vi "IR GALVO CONTROL (MULTI SPOT).vi"() -> ()   [LabVIEW 2015]
uses:
  <vilib>/DAQmx/write.llb/DAQmx Write (Analog 2D DBL NChan NSamp).vi
  <vilib>/DAQmx/configure/timing.llb/DAQmx Timing (Sample Clock).vi
  <vilib>/DAQmx/miscellaneous.llb/DAQmx Fill In Error Info.vi
panel:
  in  "Stop Button":bool
  in  "Cycle Time (ms)":i32=50
  in  "IR Stimulus Settings":cluster{"X":dbl, "Y":dbl, "TON (ms)":dbl}[](array[cluster])=[{"X"=600.0, "Y"=600.0, "TON (ms)"=12.5}, {"X"=1200.0, "Y"=1200.0, "TON (ms)"=12.5}, {"X"=1800.0, "Y"=1800.0, "TON (ms)"=12.5}, {"X"=2400.0, "Y"=2400.0, "TON (ms)"=12.5}] {"TON (ms)" step=0.1 format="%#.1f"; "Y" step=1.0 format="%#.0f"; "X" step=1.0 format="%#.0f"}
  in  "DAQmx Task Name":refnum<k21>="GALVO 1"
  out "Stim Count":i32
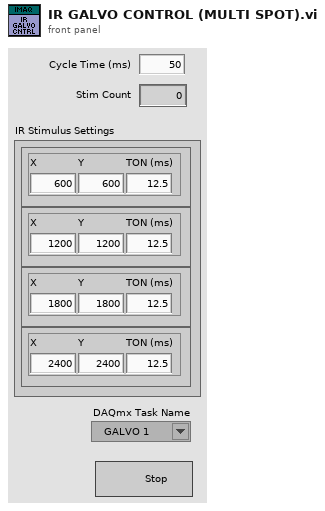
[diagram p1: front panel]
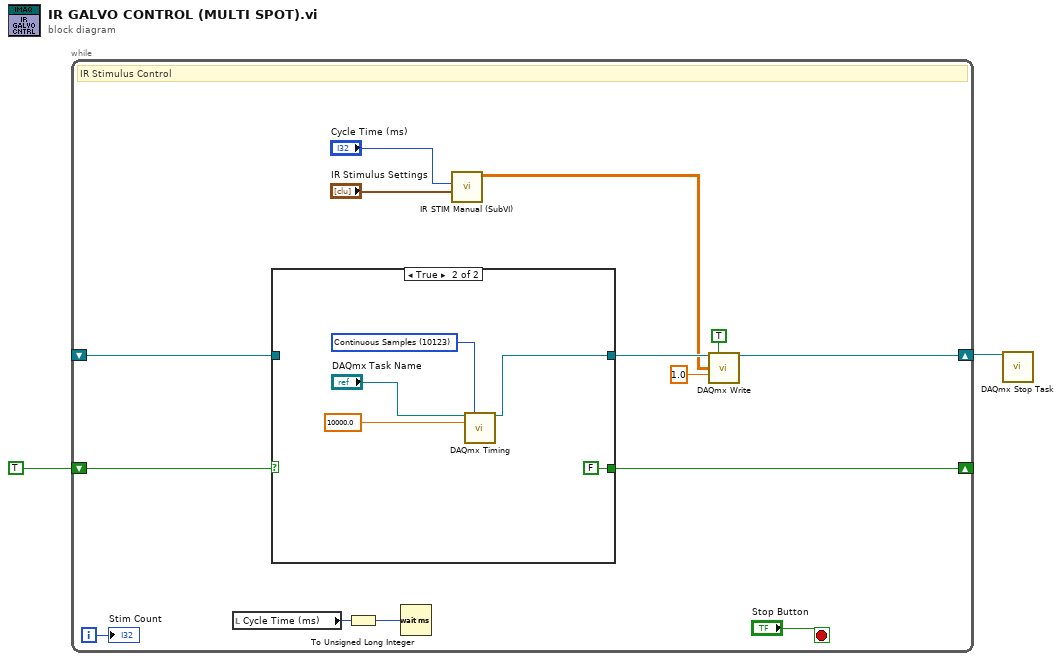
[diagram p0: block diagram]
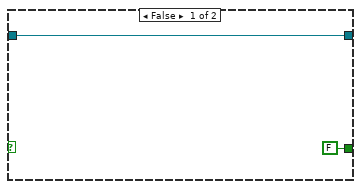
[diagram p2: hidden frame]
diagram:
  n1 = while {
    shift-right: [w12] -> w2
    shift-left: _ -> [w14]
    shift-right: [w10] -> _
    shift-left: TRUE -> [w11]
    i -> [w13]
    stop <- "Stop Button" stop-if-true
    # "IR Stimulus Control"
    n2 = local read "Cycle Time (ms)"() -> (w16:i32)
    n3 = case shown="True" w11 {
      tunnel: [FALSE FALSE] -> w10
      tunnel: w14 -> [w17 _]
      tunnel: [w17 w19] -> w6
      frame False {
      }
      frame True {
        w23 = 10123 items=["Finite Samples"=10178, "Continuous Samples"=10123, "Hardware Timed Single Point"=12522] ("sample mode")
        n4 = call-poly <vilib>:"DAQmx Timing.vi"("task/channels in"="DAQmx Task Name", "sample mode"=w23, "rate"=10000.0 ("Rate")) -> ("task out"=w19:refnum<k21>)  [unwired: 11 in, 1 out]
      }
    }
    n5 = To Unsigned Long Integer(number=w16) -> (unsigned 32bit integer=w15:u32)
    n6 = Wait (ms)(milliseconds to wait=w15) -> ()  [unwired: 1 out]
    n7 = call "IR STIM Manual (SubVI).vi"("IR Stimulus Settings"="IR Stimulus Settings", "Cycle Time (ms)"="Cycle Time (ms)") -> ("DAQ Data"=w3:dbl[][])  [unwired: 9 in]
    n8 = call-poly <vilib>:"DAQmx Write.vi"("task/channels in"=w6, "auto start"=TRUE, "data"=w3, "timeout"=1.0) -> ("task out"=w12:refnum<k21>)  [unwired: 9 in, 2 out]
    "Stim Count" <- w13
  }
  n9 = call <vilib>:"DAQmx Stop Task.vi"("task/channels in"=w2) -> ()  [unwired: 13 in, 2 out]
